vi "Get User Input.vi"(9 "Select user profile:":u16(ring) items=["test1", "test2", "test3", "test4"], 11 "Strings []":string[](array[string])) -> (1 "user":u16)   [LabVIEW 2017]
panel:
  in  "OK":bool
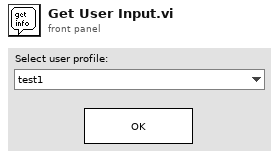
[diagram p1: front panel]
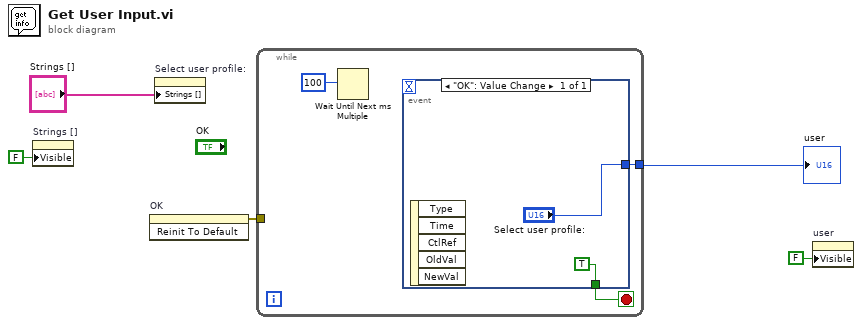
[diagram p0: block diagram]
diagram:
  n1 = property on="Strings []" class="Arr (strict)"("Visible"=FALSE) -> ()  [unwired: 2 in, 2 out]
  n2 = invoke on="OK" class="Bool" method="Reinit To Default"() -> (error out=w5:errorcluster)  [unwired: 3 in, 2 out]
  n3 = property on="Select user profile:" class="Ring (strict)"("Strings []"="Strings []") -> ()  [unwired: 2 in, 2 out]
  n4 = while {
    tunnel: [w8] -> w4
    tunnel: w5 -> [_]
    stop <- w6 stop-if-true
    n5 = Wait Until Next ms Multiple(millisecond multiple=100) -> ()  [unwired: 1 out]
    n6 = event shown="[0] \"OK\": Value Change" {
      selector: _ -> [_]
      dyn-events: _ -> [_]
      timeout: _ -> [_]
      tunnel: [TRUE] -> w6
      tunnel: ["Select user profile:"] -> w8
      event "OK": Value Change {
        n7 = event-data() -> ()  [unwired: 6 out]
      }
    }
  }
  "user" <- w4
  n8 = property on="user" class="DigNum (strict)"("Visible"=FALSE) -> ()  [unwired: 2 in, 2 out]
